vi "Main.vi"() -> ()   [LabVIEW 2021]
uses:
  <vilib>/DAQmx/write.llb/DAQmx Write (Analog DBL 1Chan 1Samp).vi
  <vilib>/DAQmx/read.llb/DAQmx Read (Analog 1D DBL 1Chan NSamp).vi
  <vilib>/Analysis/baseanly.llb/Mean (DBL).vi
  <vilib>/DAQmx/create/channels.llb/DAQmx Create Channel (AI-Voltage-Basic).vi
  <vilib>/DAQmx/configure/timing.llb/DAQmx Timing (Sample Clock).vi
  <vilib>/DAQmx/create/channels.llb/DAQmx Create Channel (AO-Voltage-Basic).vi
  <vilib>/DAQmx/miscellaneous.llb/DAQmx Fill In Error Info.vi
  <vilib>/Analysis/3filter.llb/Butterworth Filter (DBL).vi
  <vilib>/Analysis/NI_AALBase.lvlib
panel:
  out "loops":i32
  out "Log Period":dbl
  out "Samples p/channel":i32
  in  "data 2":dbl(slide) scale=-10.0..10.0
  out "Loop":i32
  out "Waveform Graph":dbl[](graph)
  out "Time elapsed":dbl
  in  "stop":bool
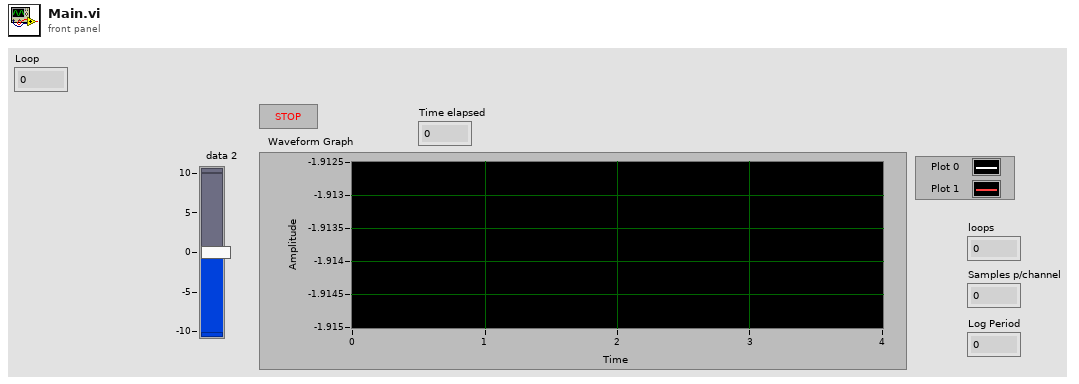
[diagram p1: front panel]
types:
  T1 = enum16{"open", "replace", "create", "open or create", "replace or create", "replace or create with confirmation"}
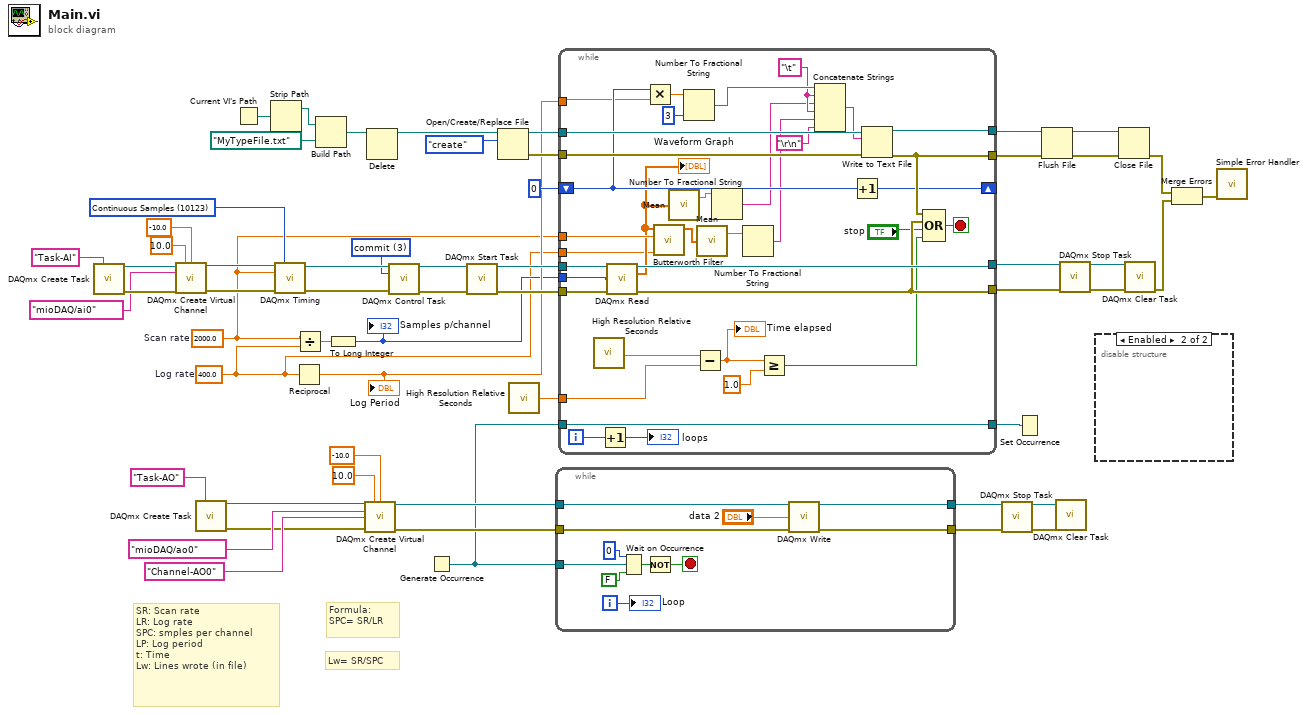
[diagram p0: block diagram]
diagram:
  w1 = 400.0  # Log rate
  w32 = 3 items=["verify"=2, "reserve"=4, "commit"=3, "unreserve"=5, "abort"=6] ("action")
  w6 = 2000.0  # Scan rate
  w38 = 10123 items=["Finite Samples"=10178, "Continuous Samples"=10123, "Hardware Timed Single Point"=12522] ("sample mode")
  # "Lw= SR/SPC"
  # "Formula:\nSPC= SR/LR"
  # "SR: Scan rate\nLR: Log rate\nSPC: smples per channel\nLP: Log period\nt: Time\nLw: Lines wrote (in file)"
  n1 = call <vilib>:"DAQmx Create Task.vi"("new task name"="Task-AI") -> ("task out"=w45:refnum<k21>, "error out"=w44:errorcluster)  [unwired: 13 in]
  n2 = call-poly <vilib>:"DAQmx Create Virtual Channel.vi"("task in"=w45, "maximum value"=10.0, "minimum value"=-10.0, "physical channels"=tag "mioDAQ/ai0", "error in"=w44) -> ("task out"=w43:refnum<k21>, "error out"=w42:errorcluster)  [unwired: 9 in]
  n3 = call <vilib>:"DAQmx Create Task.vi"("new task name"="Task-AO") -> ("task out"=w22:refnum<k21>, "error out"=w23:errorcluster)  [unwired: 13 in]
  n4 = Current VI's Path() -> (path=w12:path)
  n5 = Strip Path(path=w12) -> (stripped path=w13:path)  [unwired: 1 out]
  n6 = call-poly <vilib>:"DAQmx Timing.vi"("task/channels in"=w43, "sample mode"=w38, "rate"=w6, "error in"=w42) -> ("task out"=w47:refnum<k21>, "error out"=w46:errorcluster)  [unwired: 10 in]
  n7 = Reciprocal(x=w1) -> (1/x=w9:dbl)
  "Log Period" <- w9
  n8 = Divide(x=w6, y=w1) -> (x/y=w8:dbl)
  n9 = Build Path(base path=w13, name or relative path=path "MyTypeFile.txt") -> (appended path=w15:path)
  n10 = To Long Integer(number=w8) -> (32bit integer=w7:i32)
  "Samples p/channel" <- w7
  n11 = call-poly <vilib>:"DAQmx Create Virtual Channel.vi"("task in"=w22, "maximum value"=10.0, "minimum value"=-10.0, "physical channels"=tag "mioDAQ/ao0", "name to assign"="Channel-AO0", "error in"=w23) -> ("task out"=w24:refnum<k21>, "error out"=w25:errorcluster)  [unwired: 8 in]
  n12 = Delete(path (use dialog)=w15) -> (deleted path=w11:path)  [unwired: 4 in, 2 out]
  n13 = call <vilib>:"DAQmx Control Task.vi"("task/channels in"=w47, "action"=w32, "error in"=w46) -> ("task out"=w50:refnum<k21>, "error out"=w51:errorcluster)  [unwired: 11 in]
  n14 = Generate Occurrence() -> (w19:refnum<k4>)
  n15 = call <vilib>:"DAQmx Start Task.vi"("task/channels in"=w50, "error in"=w51) -> ("task out"=w49:refnum<k21>, "error out"=w48:errorcluster)  [unwired: 12 in]
  n16 = Open/Create/Replace File(file path (use dialog)=w11, operation (0:open)=T1."create") -> (refnum out=w55:refnum<file>, error out=w54:errorcluster)  [unwired: 4 in, 1 out]
  n17 = call <vilib>:"High Resolution Relative Seconds.vi"() -> ("relative seconds"=w33:dbl)
  n18 = while {
    tunnel: w24 -> [w68]
    tunnel: w25 -> [w67]
    tunnel: [w66] -> w26
    tunnel: [w65] -> w27
    tunnel: w19 -> [w63]
    i -> [w58]
    stop <- w59 stop-if-true
    n19 = Wait on Occurrence(1:FALSE ("ignore previous (T)"), 2:w63, 3:0 ("ms timeout (-1)")) -> (0:w60:bool)
    n20 = Not(x=w60) -> (.not. x?=w59:bool)
    n21 = call-poly <vilib>:"DAQmx Write.vi"("task/channels in"=w68, "data"="data 2", "error in"=w67) -> ("task out"=w66:refnum<k21>, "error out"=w65:errorcluster)  [unwired: 10 in, 1 out]
    "Loop" <- w58
  }
  n22 = while {
    tunnel: w55 -> [w104]
    tunnel: w54 -> [w88]
    tunnel: [w103] -> w2
    tunnel: [w99] -> w3
    tunnel: [w102] -> w53
    tunnel: [w98] -> w52
    tunnel: w49 -> [w101]
    tunnel: w48 -> [w100]
    tunnel: w33 -> [w94]
    tunnel: w19 -> [w90]
    tunnel: [w90] -> w18
    shift-right: [w89] -> _
    shift-left: 0 ("number of samples per channel") -> [w86]
    tunnel: w9 -> [w85]
    tunnel: w7 -> [w76]
    tunnel: w6 -> [w77]
    tunnel: w1 -> [w69]
    i -> [w80]
    stop <- w96 stop-if-true
    w75 = "\t" ("string")
    n23 = call <vilib>:"High Resolution Relative Seconds.vi"() -> ("relative seconds"=w95:dbl)
    n24 = Increment(x=w80) -> (x+1=→"loops":i32)
    n25 = call-poly <vilib>:"DAQmx Read.vi"("task/channels in"=w101, "number of samples per channel"=w76, "error in"=w100) -> ("task out"=w102:refnum<k21>, "data"=w71:dbl[], "error out"=w98:errorcluster)  [unwired: 10 in]
    "Waveform Graph" <- w71
    n26 = Multiply(x=w86, y=w85) -> (x*y=w87:dbl)
    n27 = call-poly <vilib>:"Butterworth Filter.vi"("low cutoff freq: fl"=w69, "sampling freq: fs"=w77, "X"=w71) -> ("Filtered X"=w78:dbl[])  [unwired: 5 in, 1 out]
    n28 = call-poly <vilib>:"Mean.vi"("X"=w71) -> ("mean"=w72:dbl)  [unwired: 1 out]
    n29 = Number To Fractional String(number=w87, precision (6)=i16 3) -> (F-format string=w83:string)  [unwired: 2 in]
    n30 = Subtract(x=w95, y=w94) -> (x-y=w93:dbl)
    "Time elapsed" <- w93
    n31 = call-poly <vilib>:"Mean.vi"("X"=w78) -> ("mean"=w81:dbl)  [unwired: 1 out]
    n32 = Number To Fractional String(number=w72) -> (F-format string=w70:string)  [unwired: 3 in]
    n33 = Number To Fractional String(number=w81) -> (F-format string=w74:string)  [unwired: 3 in]
    n34 = Greater Or Equal?(x=w93, y=1.0) -> (x >= y?=w91:bool)
    n35 = Concatenate Strings(w83, w75, w70, w75, w74, "\r\n") -> (w84:string)
    n36 = Increment(x=w86) -> (x+1=w89:i32)
    n37 = Write to Text File(file (use dialog)=w104, text=w84, error in=w88) -> (refnum out=w103:refnum<file>, error out=w99:errorcluster)  [unwired: 1 in, 1 out]
    n38 = Compound Arithmetic op=OR(w99, w98, "stop", w91) -> (w96:bool)
  }
  n39 = call <vilib>:"DAQmx Stop Task.vi"("task/channels in"=w26, "error in"=w27) -> ("task out"=w20:refnum<k21>, "error out"=w21:errorcluster)  [unwired: 12 in]
  n40 = Set Occurrence(w18) -> ()
  n41 = Flush File(refnum=w2, error in=w3) -> (refnum out=w5:refnum<file>, error out=w4:errorcluster)
  n42 = call <vilib>:"DAQmx Clear Task.vi"("task in"=w20, "error in"=w21) -> ()  [unwired: 13 in, 1 out]
  n43 = call <vilib>:"DAQmx Stop Task.vi"("task/channels in"=w53, "error in"=w52) -> ("task out"=w56:refnum<k21>, "error out"=w57:errorcluster)  [unwired: 12 in]
  n44 = disable-structure shown="Enabled" {
    frame Disabled {
    }
    frame Enabled {
    }
  }
  n45 = Close File(refnum=w5, error in=w4) -> (error out=w36:errorcluster)  [unwired: 1 out]
  n46 = call <vilib>:"DAQmx Clear Task.vi"("task in"=w56, "error in"=w57) -> ("error out"=w35:errorcluster)  [unwired: 13 in]
  n47 = Merge Errors(w36, w35) -> (w37:errorcluster)
  n48 = call <vilib>:"Simple Error Handler.vi"("error in (no error)"=w37) -> ()  [unwired: 4 in, 5 out]
